vi "WGP2.vi"() -> ()   [LabVIEW 2017]
doc: "Warren Green\nPhysics 350\n\nThis program collects and graphs data on the top graph, while also graphing the average. \nThe bottom graph displays the averaged data and then allows the user to estamate a more precises fit over the average.\nThe user also has the option to save the data or reset the graph."
uses:
  P2B sol/typedefs/measurement parameters.ctl
  P2B sol/typedefs/ferro response parameter cluster.ctl
panel:
  in  "reset":bool
  in  "Stop":bool
  in  "Save Data":bool
  out "Data to Save":dbl[][](array[numeric]) format="%#_4g"
  in  "Fitting Parameters":T1={"amplitude a (V)"=5.0, "time const a (uS)"=15.0, "amplitude b (V)"=10.0, "time const b (uS)"=150.0} {"time const b (uS)" scale=0.0..200.0; "amplitude b (V)" scale=0.0..50.0; "time const a (uS)" scale=0.0..200.0; "amplitude a (V)" scale=0.0..50.0}
  out "Analysis Graph":T2(graph)
  out "Acquisition Graph":T3(graph)
  out "count":i32
  in  "Meas Params":T4={"time step (uS)"=1.0, "N meas"=1000, "N meas reps"=100} caption="Measurement Parameters"
  in  "Start":bool
  # "Simulated FerroElectric Experiment"
  # "Warren Green\nPhysics 350"
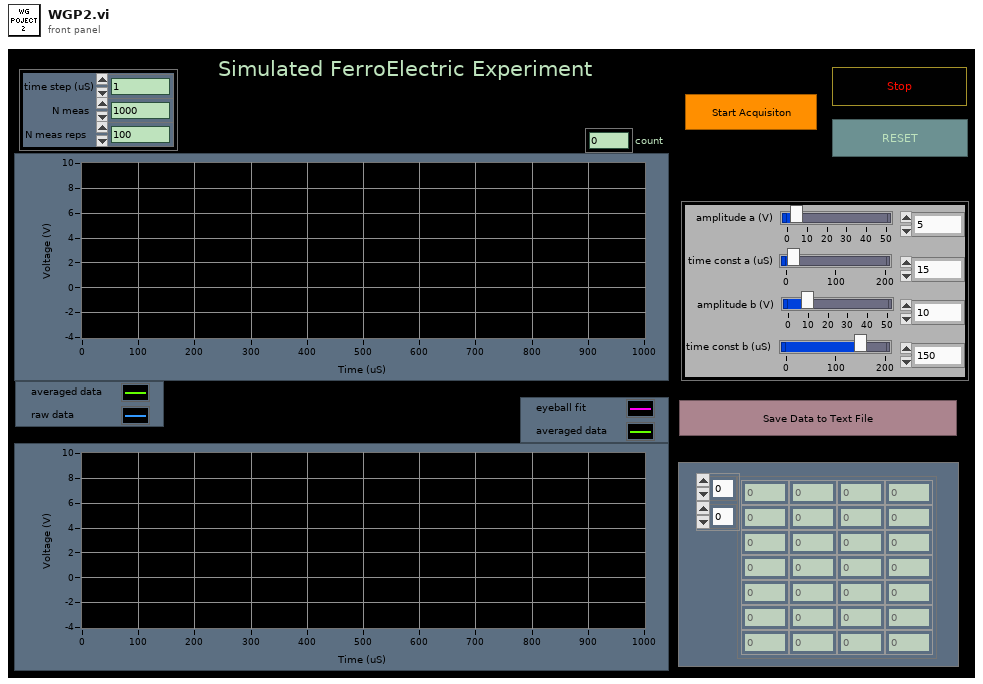
[diagram p1: front panel]
types:
  T1 = typedef "ferro response parameter cluster.ctl" = cluster{"amplitude a (V)":dbl, "time const a (uS)":dbl, "amplitude b (V)":dbl, "time const b (uS)":dbl}
  T2 = cluster{"time array (uS)":dbl[], "voltage array out (V)":dbl[]}[]
  T3 = cluster{"time array (s)":dbl[], "voltage array (V)":dbl[]}[]
  T4 = typedef "measurement parameters.ctl" = cluster{"time step (uS)":dbl, "N meas":i32, "N meas reps":i32}
  T5 = cluster{"time array (s)":dbl[], "voltage array (V)":dbl[]}
  T6 = cluster{"time array out (uS)":dbl[], "voltage array out (V)":dbl[]}
  T7 = cluster{"time array (s)":dbl[], "voltage array out (V)":dbl[]}[]
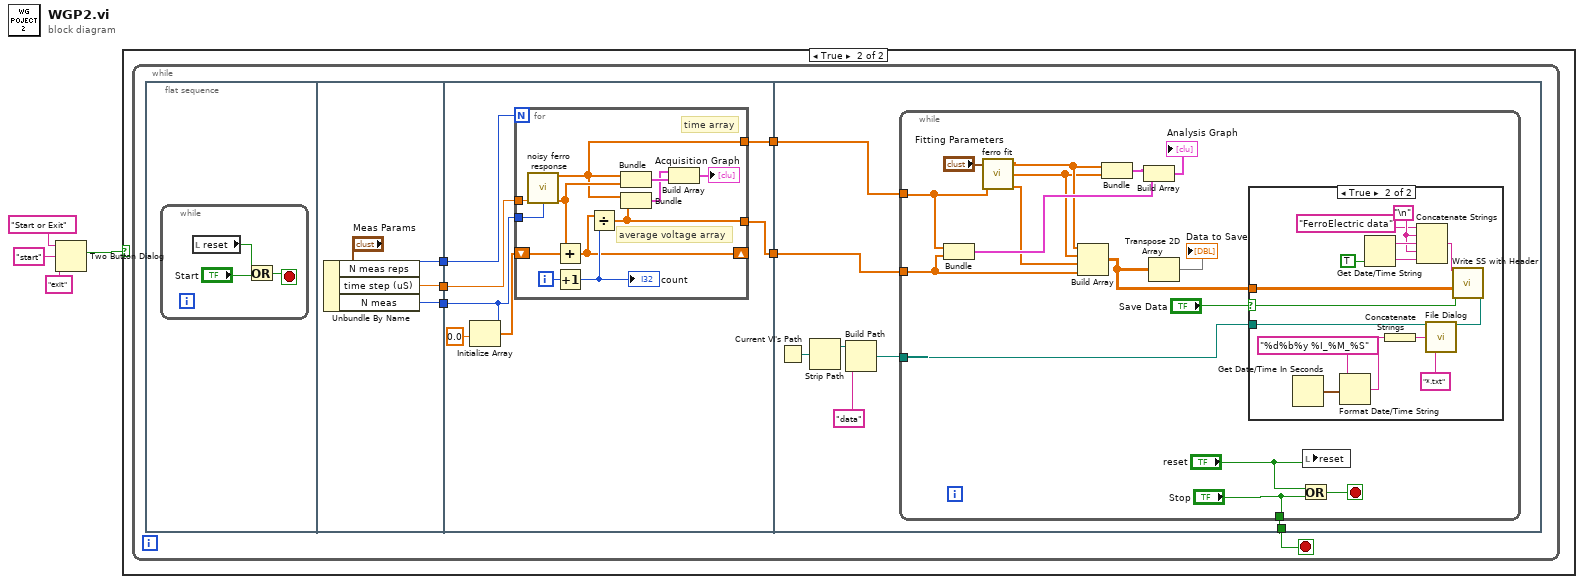
[diagram p0: block diagram]
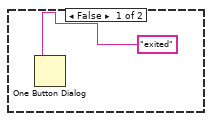
[diagram p2: hidden frame]
diagram:
  n1 = Two Button Dialog(message="Start or Exit", 1:"exit", 2:"start") -> (T button?=w1:bool)
  n2 = case shown="True" w1 {
    frame False {
      n3 = One Button Dialog(message="exited") -> ()  [unwired: 1 in, 1 out]
    }
    frame True {
      n4 = while {
        stop <- w6 stop-if-true
        n5 = flat-sequence {
          tunnel: [w17] -> w11
          tunnel: [w16] -> w10
          tunnel: [w15] -> w9
          tunnel: w11 -> [w21]
          tunnel: w10 -> [w23]
          tunnel: w9 -> [w22]
          tunnel: [w20] -> w8
          tunnel: [w19] -> w7
          tunnel: w8 -> [w43]
          tunnel: w7 -> [w44]
          tunnel: [w38] -> w6
          frame #0 {
            n6 = while {
              stop <- w12 stop-if-true
              n7 = local read "reset"() -> (w14:bool)
              n8 = Or(x=w14, y="Start") -> (x .or. y?=w12:bool)
            }
          }
          frame #1 {
            n9 = Unbundle By Name("Meas Params") -> ("N meas reps"=w15:i32, "time step (uS)"=w17:dbl, "N meas"=w16:i32)
          }
          frame #2 {
            n10 = Initialize Array(0.0 ("element"), w23) -> (w25:dbl[])
            n11 = for {
              N: w22 -> [_]
              tunnel: w21 -> [w37]
              tunnel: w23 -> [w36]
              shift-right: [w30] -> _
              shift-left: w25 -> [w31]
              tunnel: [w27] -> w20
              tunnel: [w26] -> w19
              i -> [w35]
              # "average voltage array"
              # "time array"
              n12 = call "noisy ferro response.vi"("time step (uS)"=w37, "N meas"=w36) -> ("time array (s)"=w27:dbl[], "voltage array (V)"=w32:dbl[])  [unwired: 12 in]
              n13 = Add(x=w32, y=w31) -> (x+y=w30:dbl[])
              n14 = Increment(x=w35) -> (x+1=w34:i32)
              "count" <- w34
              n15 = Divide(x=w30, y=w34) -> (x/y=w26:dbl[])
              n16 = Bundle("time array (s)"=w27, "voltage array (V)"=w32) -> (w29:T5)  [unwired: 1 in]
              n17 = Bundle("time array (s)"=w27, w26) -> (w28:cluster{"time array (s)":dbl[], dbl[]})  [unwired: 1 in]
              n18 = Build Array(w28, w29) -> (→"Acquisition Graph":T3)
            }
          }
          frame #3 {
            n19 = Current VI's Path() -> (path=w42:path)
            n20 = Strip Path(path=w42) -> (stripped path=w39:path)  [unwired: 1 out]
            n21 = Build Path(base path=w39, name or relative path="data") -> (appended path=w40:path)
            n22 = while {
              tunnel: w43 -> [w54]
              tunnel: w44 -> [w53]
              tunnel: w40 -> [w49]
              tunnel: ["Stop"] -> w38
              stop <- w46 stop-if-true
              n23 = Bundle("time array (s)"=w54, w53) -> (w58:cluster{"time array (s)":dbl[], dbl[]})  [unwired: 1 in]
              n24 = call "ferro fit.vi"("ferro response parameters"="Fitting Parameters", "time array in (uS)"=w54) -> ("parameters array out"=w52:dbl[], "voltage array out (V)"=w50:dbl[], "time array out (uS)"=w51:dbl[])  [unwired: 7 in]
              n25 = Build Array(w51, w50, w52, w53) -> (w48:dbl[][])
              n26 = Bundle("time array out (uS)"=w51, "voltage array out (V)"=w50) -> (w59:T6)  [unwired: 1 in]
              n27 = Build Array(w59, w58) -> (→"Analysis Graph":T7)
              n28 = Transpose 2D Array(2D array=w48) -> (transposed array=→"Data to Save":dbl[][])
              n29 = case shown="True" "Save Data" {
                selector: "Save Data" -> [_ w74]
                tunnel: w48 -> [_ w75]
                tunnel: w49 -> [_ w66]
                frame False {
                }
                frame True {
                  w70 = "\n"
                  n30 = Get Date/Time In Seconds() -> (seconds since 1Jan1904=w63:timestamp)
                  n31 = Format Date/Time String(time format string (%c)="%d%b%y %I_%M_%S", seconds (now)=w63) -> (date/time string=w62:string)  [unwired: 1 in]
                  n32 = Get Date/Time String(want seconds? (F)=TRUE) -> (date string=w71:string, time string=w72:string)  [unwired: 2 in]
                  n33 = Concatenate Strings(w62) -> (w64:string)
                  n34 = Concatenate Strings("FerroElectric data" ("Header String"), w70, w71, w70, w72) -> (w68:string)
                  n35 = call "File Dialog"("start path"=w66, "default name"=w64, "pattern (all files)"="*.txt") -> ("selected path"=w65:path)  [unwired: 9 in, 3 out]
                  n36 = call "Write SS with Header.vi"("Header String"=w68, "Data to Write"=w75, "Transpose Data?"=w74, "Path"=w65) -> ()  [unwired: 12 in]
                }
              }
              n37 = Or(x="reset", y="Stop") -> (x .or. y?=w46:bool)
              n38 = local write "reset"("reset") -> ()
            }
          }
        }
      }
    }
  }
